vi "Release Notifier.vi"(8 "error in (no error)":errorcluster, 10 "force destroy? (F)":bool, 11 "CVT_I32 in":refnum<class "CVT_I32.lvclass">) -> (0 "error out":errorcluster, 3 "CVT_I32 out":refnum<class "CVT_I32.lvclass">)   [LabVIEW 2024, in "Current Value Table.lvlib" / "CVT_I32.lvclass"]
uses:
  CVT_I32.lvclass
  CVT_I32.lvclass/CVT_I32.ctl
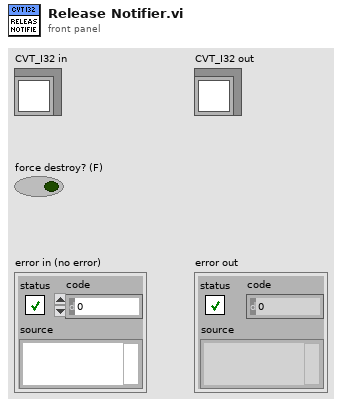
[diagram p1: front panel]
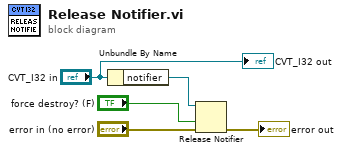
[diagram p0: block diagram]
diagram:
  n1 = Unbundle By Name("CVT_I32 in") -> ("notifier"=w4:refnum<notifier>)
  n2 = Release Notifier(notifier=w4, force destroy? (F)="force destroy? (F)", error in (no error)="error in (no error)") -> (error out=→"error out":errorcluster)  [unwired: 2 out]
  "CVT_I32 out" <- "CVT_I32 in"
